vi "main.vi"() -> ()   [LabVIEW 2021]
uses:
  student.ctl
panel:
  in  "stop":bool
  in  "Update":bool
  in  "student 3":T1
  out "student 2":T1
  out "Dane Wejœciowe":T1[](array[typedef])
  in  "Indeks":i32
  out "student":T1
  in  "Idx":i32
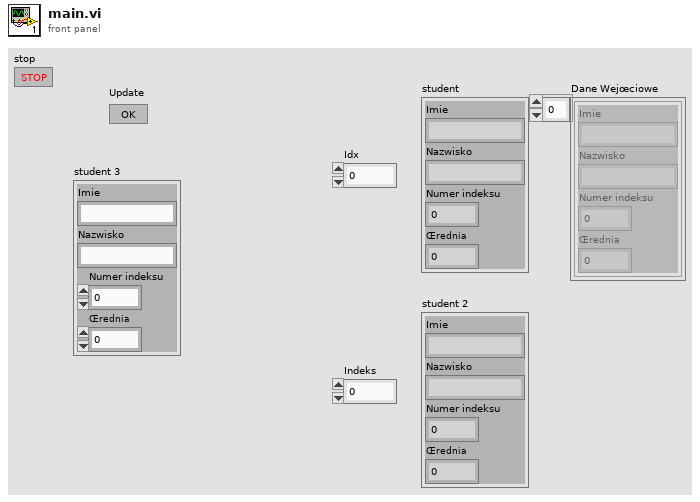
[diagram p1: front panel]
types:
  T1 = typedef "student.ctl" = cluster{"Imie":string, "Nazwisko":string, "Numer indeksu":i32, "Œrednia":dbl}
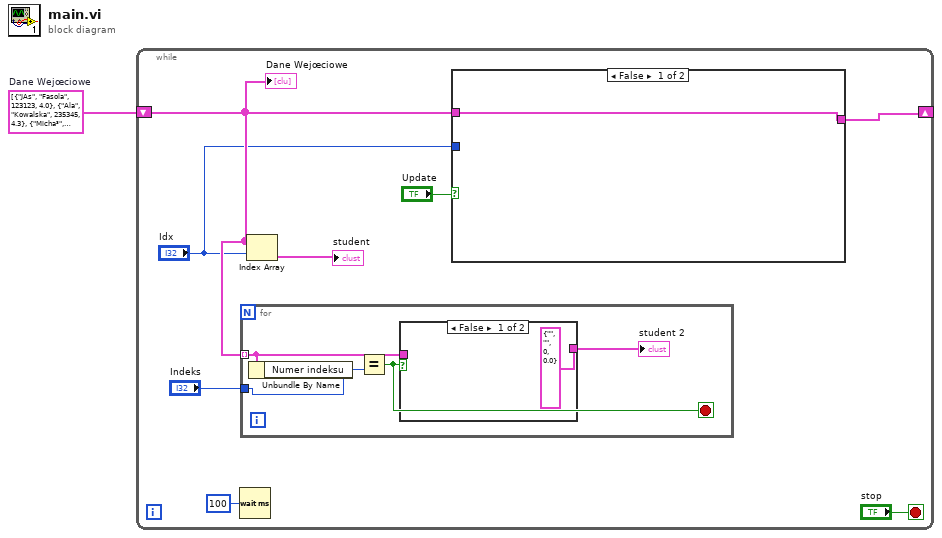
[diagram p0: block diagram]
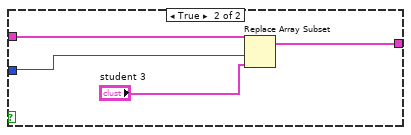
[diagram p2: hidden frame]
diagram:
  w1 = T1[] [{"Imie"="JAs", "Nazwisko"="Fasola", "Numer indeksu"=123123, "Œrednia"=4.0}, {"Imie"="Ala", "Nazwisko"="Kowalska", "Numer indeksu"=235345, "Œrednia"=4.3}, {"Imie"="Micha³", "Nazwisko"="Kwiatkowski", "Numer indeksu"=2344, "Œrednia"=3.5}]  # Dane Wejœciowe
  n1 = while {
    shift-right: [w3] -> _
    shift-left: w1 -> [w5]
    stop <- "stop" stop-if-true
    n2 = Wait (ms)(milliseconds to wait=u32 100) -> ()  [unwired: 1 out]
    n3 = for {
      tunnel: w5 -> [w16] mode=indexing
      tunnel: "Indeks" -> [w18]
      stop <- w15 stop-if-true
      n4 = Unbundle By Name(w16) -> ("Numer indeksu"=w19:i32)
      n5 = Equal?(x=w19, y=w18) -> (x = y?=w15:bool)
      n6 = case shown="False" w15 {
        tunnel: [T1 {"Imie"="", "Nazwisko"="", "Numer indeksu"=0, "Œrednia"=0.0} w21] -> w17
        tunnel: w16 -> [_ w21]
        frame False {
        }
        frame True {
        }
      }
      "student 2" <- w17
    }
    n7 = Index Array(array=w5, index="Idx") -> (element=→"student":T1)
    n8 = case shown="False" "Update" {
      tunnel: w5 -> [w10 w14]
      tunnel: "Idx" -> [_ w13]
      tunnel: [w10 w11] -> w3
      frame False {
      }
      frame True {
        n9 = Replace Array Subset(array=w14, new element="student 3", index=w13) -> (w11:T1[])
      }
    }
    "Dane Wejœciowe" <- w5
  }
